vi "Example TCP Client-Server.vi"() -> ()   [LabVIEW 2013]
uses:
  Connection/Connection.lvclass
  Connection.TCP/Connection.TCP.lvclass
panel:
  out "server connected":bool
  out "client connected":bool
  out "Comm OK":bool
  out "value":dbl
  out "listener error":errorcluster
  out "client session error":errorcluster
  out "server session error":errorcluster
  out "Bytes":u8[](array[numeric]) format="%08b"
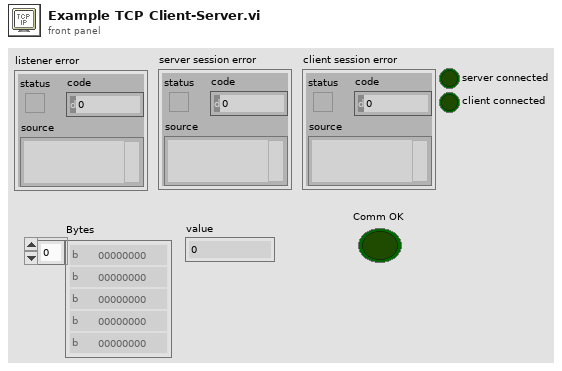
[diagram p1: front panel]
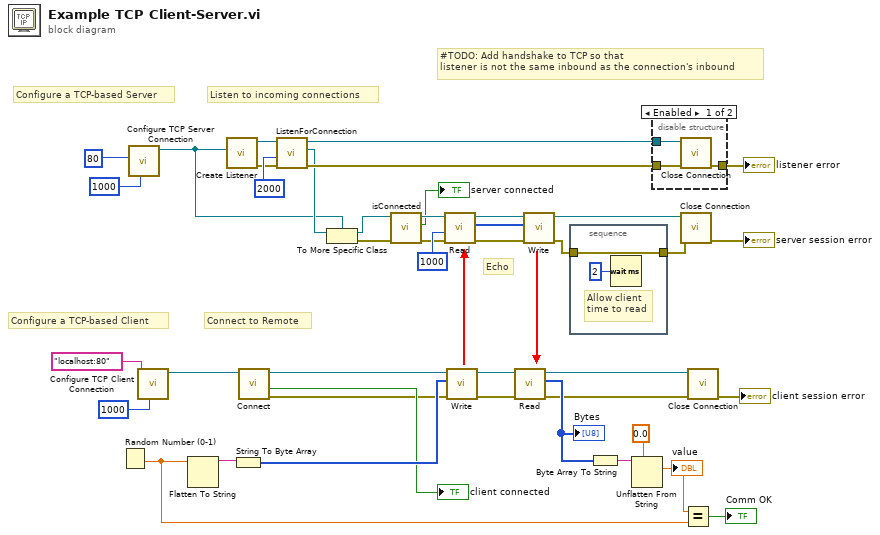
[diagram p0: block diagram]
diagram:
  # "#TODO: Add handshake to TCP so that\nlistener is not the same inbound as the connection's inbound"
  # "Configure a TCP-based Client"
  # "Connect to Remote"
  # "Echo"
  # "Listen to incoming connections"
  # "Configure a TCP-based Server"
  n1 = Random Number (0-1)() -> (number: 0 to 1=w17:dbl)
  n2 = call "Configure TCP Server Connection.vi"("timeout (5000ms)"=1000, "remote port (80)"=u16 80) -> ("Connection.TCP"=w2:refnum<class "Connection.TCP.lvclass">)  [unwired: 8 in, 1 out]
  n3 = call "Configure TCP Client Connection.vi"("timeout (5000ms)"=1000, "Authority (localhost:80)"="localhost:80" ("address (localhost)")) -> ("Connection.TCP"=w20:refnum<class "Connection.TCP.lvclass">)  [unwired: 8 in, 1 out]
  n4 = Flatten To String(anything=w17) -> (data string=w30:string)  [unwired: 3 in, 2 out]
  n5 = call "Create Listener.vi"("Connection Configuration"=w2) -> ("error out"=w39:errorcluster, "Listener"=w42:refnum<class "Connection.lvclass">)  [unwired: 9 in]
  n6 = String To Byte Array(string=w30) -> (unsigned byte array=w29:u8[])
  n7 = call "Connect.vi"("Connection in"=w20) -> ("error out"=w8:errorcluster, "Connection Established"=→"client connected":bool, "Connection out"=w9:refnum<class "Connection.TCP.lvclass">)  [unwired: 8 in]
  n8 = call "ListenForConnection.vi"("error in (no error)"=w39, "timeout (2000 ms)"=2000 ("bytes to read (100)"), "Listener"=w42) -> ("error out"=w24:errorcluster, "Connection"=w6:refnum<class "Connection.lvclass">, "Listener out"=w40:refnum<class "Connection.lvclass">)  [unwired: 5 in, 1 out]
  n9 = To More Specific Class(target class=w2, reference=w6) -> (specific class reference=w5:refnum<class "Connection.TCP.lvclass">, error out=w4:errorcluster)  [unwired: 1 in]
  n10 = call "isConnected.vi"("error in (no error)"=w4, "Connection in"=w5) -> ("error out"=w12:errorcluster, "connected"=→"server connected":bool, "Connection out"=w13:refnum<class "Connection.TCP.lvclass">)  [unwired: 7 in]
  n11 = call "Read.vi"("error in (no error)"=w12, "timeout (2000 ms)"=1000 ("bytes to read (100)"), "TCPConnection in"=w13) -> ("error out"=w34:errorcluster, "Bytes"=w36:u8[], "TCPConnection out"=w37:refnum<class "Connection.TCP.lvclass">)  [unwired: 4 in, 2 out]
  n12 = call "Write.vi"("error in (no error)"=w8, "Bytes"=w29, "Connection in"=w9) -> ("error out"=w33:errorcluster, "Connection"=w35:refnum<class "Connection.TCP.lvclass">)  [unwired: 6 in, 1 out]
  n13 = call "Read.vi"("error in (no error)"=w33, "TCPConnection in"=w35) -> ("error out"=w22:errorcluster, "Bytes"=w28:u8[], "TCPConnection out"=w21:refnum<class "Connection.TCP.lvclass">)  [unwired: 5 in, 2 out]
  "Bytes" <- w28
  n14 = call "Write.vi"("error in (no error)"=w34, "Bytes"=w36, "Connection in"=w37) -> ("error out"=w15:errorcluster, "Connection"=w31:refnum<class "Connection.TCP.lvclass">)  [unwired: 6 in, 1 out]
  n15 = stacked-sequence {
    tunnel: w15 -> [w43]
    tunnel: [w43] -> w14
    frame #0 {
      # "Allow client\ntime to read"
      n16 = Wait (ms)(milliseconds to wait=u32 2) -> ()  [unwired: 1 out]
    }
  }
  n17 = Byte Array To String(unsigned byte array=w28) -> (string=w27:string)
  n18 = Unflatten From String(type=0.0, binary string=w27) -> (value=w18:dbl)  [unwired: 3 in, 2 out]
  "value" <- w18
  n19 = disable-structure shown="Enabled" {
    disable-tunnel: w40 -> [w47 _]
    disable-tunnel: w24 -> [w46 w48]
    disable-tunnel: [w45 w48] -> w23
    frame Enabled {
      n20 = call "Close Connection.vi"("error in (no error)"=w46, "Connection in"=w47) -> ("error out"=w45:errorcluster)  [unwired: 8 in, 1 out]
    }
    frame Disabled {
    }
  }
  "listener error" <- w23
  n21 = call "Close Connection.vi"("error in (no error)"=w14, "Connection in"=w31) -> ("error out"=→"server session error":errorcluster)  [unwired: 8 in, 1 out]
  n22 = Equal?(x=w18, y=w17) -> (x = y?=→"Comm OK":bool)
  n23 = call "Close Connection.vi"("error in (no error)"=w22, "Connection in"=w21) -> ("error out"=→"client session error":errorcluster)  [unwired: 8 in, 1 out]
